vi "Configure Session.vi"(8 "error in":errorcluster, 11 "Plugin in":refnum<class "StreamWriter.lvclass">) -> (0 "error out":errorcluster, 3 "Plugin out":refnum<class "StreamWriter.lvclass">)   [LabVIEW 2024, in "StreamWriter.lvlib" / "StreamWriter.lvclass"]
uses:
  StreamWriter.lvclass
  C:/Program Files/National Instruments/LabVIEW 2024/vi.lib/FlexLogger/SDK/PluginSDK.lvlibp/PEFClasses/SDK/Plugin/Plugin.lvclass
  StreamWriter Parameters.ctl
  StreamWriter.lvclass/StreamWriter.ctl
  StreamWriter Strings.vi
  <vilib>/FlexLogger/SDK/PluginSDK.lvlibp/PEFClasses/SDK/Plugin/ParameterAccess/Read String.vi
  <vilib>/FlexLogger/SDK/PluginSDK.lvlibp/PEFClasses/SDK/Plugin/ParameterAccess/Read I32.vi
  <vilib>/FlexLogger/SDK/PluginSDK.lvlibp/PEFClasses/SDK/Plugin/Plugin.lvclass
  C:/Program Files/National Instruments/LabVIEW 2024/vi.lib/FlexLogger/SDK/PluginSDK.lvlibp/PEFClasses/SDK/Processing Element/Processing Element.lvclass
  C:/dev/niflexlogger-plugins/plugins/StreamWriter/source/StreamWriter/StreamWriter.lvclass
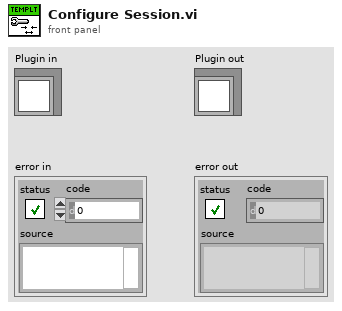
[diagram p1: front panel]
types:
  T1 = typedef "StreamWriter.lvlib/StreamWriter.lvclass/StreamWriter Parameters.ctl" = cluster{"Writer URL":string, "Buffer Size":i32, "Writer Endpoint":refnum<k21>, "Stream Names":string[]}
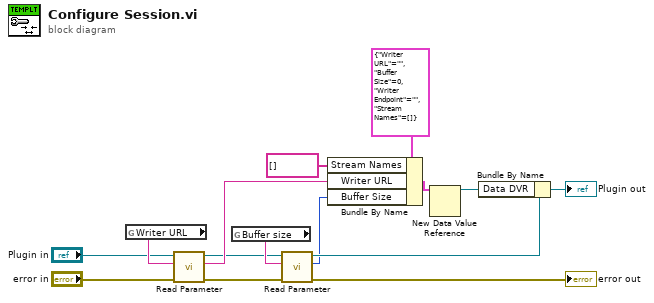
[diagram p0: block diagram]
diagram:
  n1 = global read "StreamWriter Strings.vi" "Writer URL"() -> (w7:string)
  n2 = call-poly <vilib>:"Read Parameter.vi"("error in (no error)"="error in", "Name"=w7, "Plugin in"="Plugin in") -> ("error out"=w2:errorcluster, "Value"=w4:string, "Plugin out"=w3:refnum<class "StreamWriter.lvclass">)  [unwired: 5 in, 1 out]
  n3 = global read "StreamWriter Strings.vi" "Buffer size"() -> (w9:string)
  n4 = call-poly <vilib>:"Read Parameter.vi"("error in (no error)"=w2, "Name"=w9, "Plugin in"=w3) -> ("error out"=→"error out":errorcluster, "Value"=w8:i32, "Plugin out"=w13:refnum<class "StreamWriter.lvclass">)  [unwired: 5 in, 1 out]
  n5 = Bundle By Name(cluster=T1 {"Writer URL"="", "Buffer Size"=0, "Writer Endpoint"="", "Stream Names"=[]} ("StreamWriter Parameters"), "Stream Names"=string[] [], "Writer URL"=w4, "Buffer Size"=w8) -> (w15:T1)
  n6 = New Data Value Reference(data value=w15) -> (data value reference=w12:refnum<data-value>)  [unwired: 1 in, 1 out]
  n7 = Bundle By Name(cluster=w13, "Data DVR"=w12) -> (→"Plugin out":refnum<class "StreamWriter.lvclass">)
